vi "RP Test Scale.vi"() -> ()   [LabVIEW 2024]
uses:
  RP Calibration.ctl
  RP Calibration 4ch.ctl
  RP Channel Calibration.ctl
  RP Filter 4ch.ctl
  RP Channel Filter.ctl
  RP Calibration 2ch.ctl
panel:
  out "Scaled raw":dbl[][](graph)
  out "Unscaled":i16[][](graph)
  in  "ADC scale":dbl=8192.0
  out "Scaled":dbl[][](graph)
  in  "Channels":string[](array[string])=["V0", "V1"]
  in  "Unscaled data file":path=path "C:/Data/November_2024/111824/p004_111824.tdms"
  in  "RP Calibration":T1={"dataStructureId"=5, "wpCheck"=7, "fast_adc_count_1_1"=2, "padding"=0, "fast_adc_1_1"={"ch_0"={"baseScale"=1.0, "calibValue"=2837815, "offset"=-112, "padding 2"=0, "gainCalc"=1.0571686893755443}, "ch_1"={"baseScale"=1.0, "calibValue"=2835253, "offset"=-164, "padding 2"=0, "gainCalc"=1.056214269801971}, "ch_2"={"baseScale"=0.0, "calibValue"=0, "offset"=0, "padding 2"=0, "gainCalc"=0.0}, "ch_3"={"baseScale"=0.0, "calibValue"=0, "offset"=0, "padding 2"=0, "gainCalc"=0.0}}, "fast_adc_filter_1_1"={"ch_0"={"aa"=32147, "bb"=276423, "pp"=9830, "kk"=14260634}, "ch_1"={"aa"=32147, "bb"=276423, "pp"=9830, "kk"=14260634}, "ch_2"={"aa"=0, "bb"=0, "pp"=0, "kk"=0}, "ch_3"={"aa"=0, "bb"=0, "pp"=0, "kk"=0}}, "fast_adc_count_1_20"=2, "fast_adc_1_20"={"ch_0"={"baseScale"=1.0, "calibValue"=2666775, "offset"=-152, "padding 2"=0, "gainCalc"=0.9934513108181707}, "ch_1"={"baseScale"=1.0, "calibValue"=2664836, "offset"=-221, "padding 2"=0, "gainCalc"=0.9927289768786084}, "ch_2"={"baseScale"=0.0, "calibValue"=0, "offset"=0, "padding 2"=0, "gainCalc"=0.0}, "ch_3"={"baseScale"=0.0, "calibValue"=0, "offset"=0, "padding 2"=0, "gainCalc"=0.0}}, "fast_adc_filter_1_20"={"ch_0"={"aa"=16901, "bb"=193419, "pp"=9830, "kk"=14260634}, "ch_1"={"aa"=16901, "bb"=193419, "pp"=9830, "kk"=14260634}, "ch_2"={"aa"=0, "bb"=0, "pp"=0, "kk"=0}, "ch_3"={"aa"=0, "bb"=0, "pp"=0, "kk"=0}}, "fast_adc_count_1_1_ac"=0, "fast_adc_1_1_ac"={"ch_0"={"baseScale"=0.0, "calibValue"=0, "offset"=0, "padding 2"=0, "gainCalc"=0.0}, "ch_1"={"baseScale"=0.0, "calibValue"=0, "offset"=0, "padding 2"=0, "gainCalc"=0.0}, "ch_2"={"baseScale"=0.0, "calibValue"=0, "offset"=0, "padding 2"=0, "gainCalc"=0.0}, "ch_3"={"baseScale"=0.0, "calibValue"=0, "offset"=0, "padding 2"=0, "gainCalc"=0.0}}, "fast_adc_count_1_20_ac"=0, "fast_adc_1_20_ac"={"ch_0"={"baseScale"=0.0, "calibValue"=0, "offset"=0, "padding 2"=0, "gainCalc"=0.0}, "ch_1"={"baseScale"=0.0, "calibValue"=0, "offset"=0, "padding 2"=0, "gainCalc"=0.0}, "ch_2"={"baseScale"=0.0, "calibValue"=0, "offset"=0, "padding 2"=0, "gainCalc"=0.0}, "ch_3"={"baseScale"=0.0, "calibValue"=0, "offset"=0, "padding 2"=0, "gainCalc"=0.0}}, "fast_dac_count_x1"=2, "fast_dac_x1"={"ch_0"={"baseScale"=1.0, "calibValue"=2383506, "offset"=-287, "padding 2"=0, "gainCalc"=0.8879253630482418}, "ch_1"={"baseScale"=1.0, "calibValue"=2376551, "offset"=-279, "padding 2"=0, "gainCalc"=0.8853344231051493}}, "fast_dac_count_x5"=0, "fast_dac_x5"={"ch_0"={"baseScale"=0.0, "calibValue"=0, "offset"=0, "padding 2"=0, "gainCalc"=0.0}, "ch_1"={"baseScale"=0.0, "calibValue"=0, "offset"=0, "padding 2"=0, "gainCalc"=0.0}}}
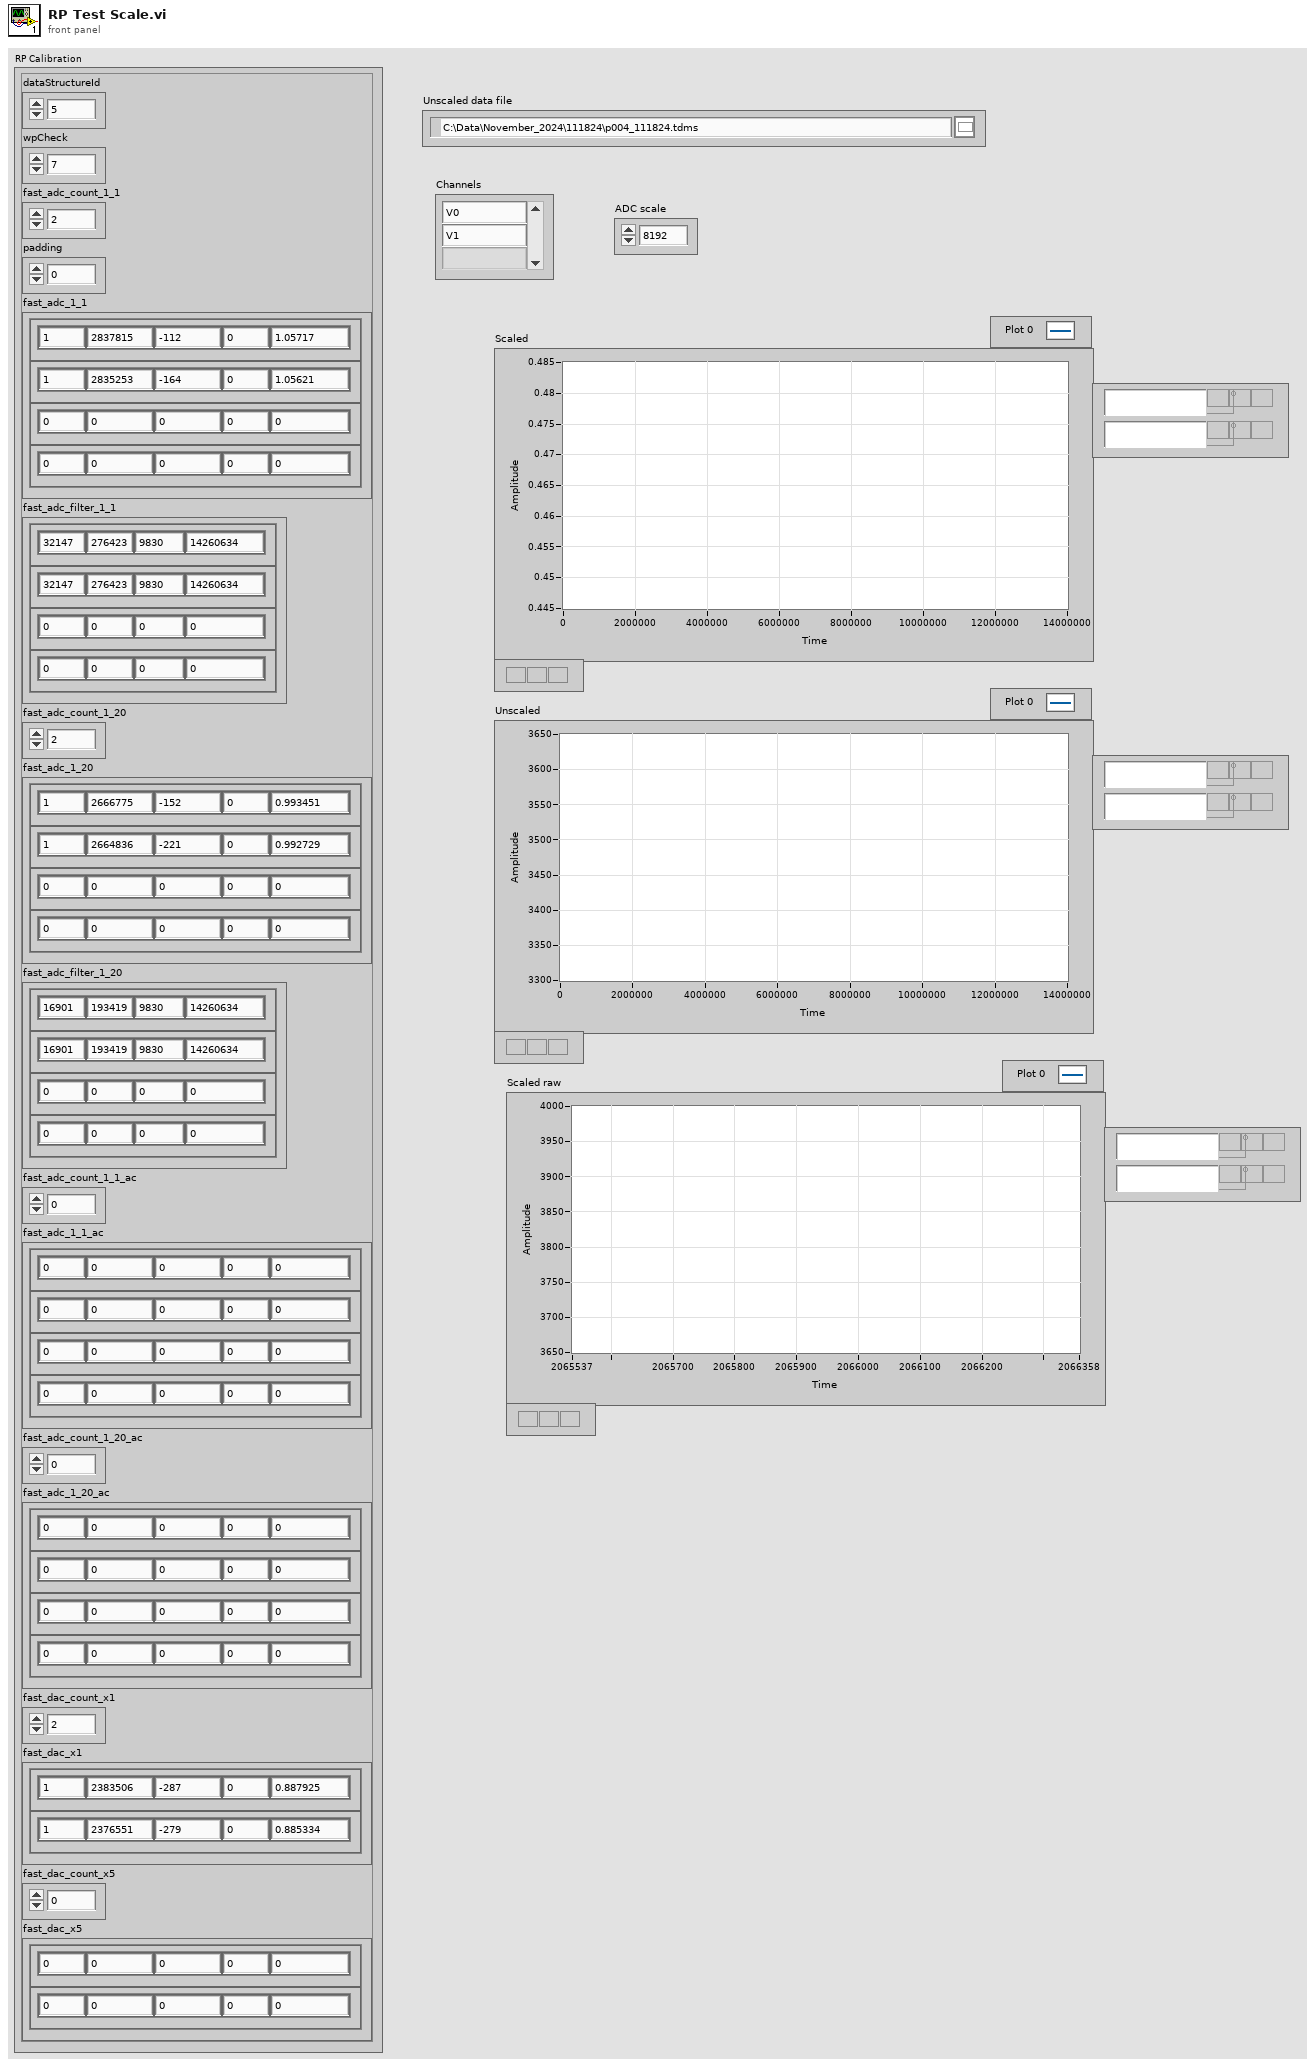
[diagram p1: front panel]
types:
  T1 = typedef "RP Calibration.ctl" = cluster{"dataStructureId":u8, "wpCheck":u8, "fast_adc_count_1_1":u16, "padding":u32, "fast_adc_1_1":T2, "fast_adc_filter_1_1":T4, "fast_adc_count_1_20":u64, "fast_adc_1_20":T2, "fast_adc_filter_1_20":T4, "fast_adc_count_1_1_ac":u64, "fast_adc_1_1_ac":T2, "fast_adc_count_1_20_ac":u64, "fast_adc_1_20_ac":T2, "fast_dac_count_x1":u64, "fast_dac_x1":T6, "fast_dac_count_x5":u64, "fast_dac_x5":T6}
  T2 = typedef "RP Calibration 4ch.ctl" = cluster{"ch_0":T3, "ch_1":T3, "ch_2":T3, "ch_3":T3}
  T3 = typedef "RP Channel Calibration.ctl" = cluster{"baseScale":sgl, "calibValue":u32, "offset":i32, "padding 2":i32, "gainCalc":dbl}
  T4 = typedef "RP Filter 4ch.ctl" = cluster{"ch_0":T5, "ch_1":T5, "ch_2":T5, "ch_3":T5}
  T5 = typedef "RP Channel Filter.ctl" = cluster{"aa":u32, "bb":u32, "pp":u32, "kk":u32}
  T6 = typedef "RP Calibration 2ch.ctl" = cluster{"ch_0":T3, "ch_1":T3}
  T7 = enum16{"open", "open or create", "create or replace", "create", "open (read-only)"}
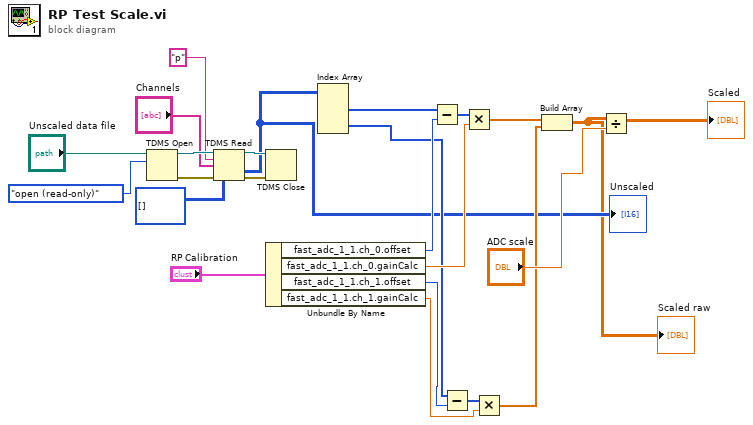
[diagram p0: block diagram]
diagram:
  n1 = TDMS Open(10:T7."open (read-only)" ("operation (0:open)"), 11:"Unscaled data file") -> (0:w21:errorcluster, 3:w22:refnum<k34>)  [unwired: 5 in]
  n2 = TDMS Read(0:w22, 5:"p" ("group name in"), 7:"Channels", 11:w21, 12:i16[][] []) -> (4:w17:refnum<k34>, 10:w2:i16[][], 15:w18:errorcluster)  [unwired: 3 in, 3 out]
  "Unscaled" <- w2
  n3 = TDMS Close(8:w18, 11:w17) -> ()  [unwired: 2 out]
  n4 = Unbundle By Name("RP Calibration") -> ("fast_adc_1_1.ch_0.offset"=w13:i32, "fast_adc_1_1.ch_0.gainCalc"=w11:dbl, "fast_adc_1_1.ch_1.offset"=w5:i32, "fast_adc_1_1.ch_1.gainCalc"=w4:dbl)
  n5 = Index Array(array=w2) -> (element #1=w14:i16[], element #2=w6:i16[])  [unwired: 4 in]
  n6 = Subtract(x=w14, y=w13) -> (x-y=w12:i32[])
  n7 = Subtract(x=w6, y=w5) -> (x-y=w7:i32[])
  n8 = Multiply(x=w12, y=w11) -> (x*y=w10:dbl[])
  n9 = Multiply(x=w7, y=w4) -> (x*y=w3:dbl[])
  n10 = Build Array(w10, w3) -> (w1:dbl[][])
  "Scaled raw" <- w1
  n11 = Divide(x=w1, y="ADC scale") -> (x/y=→"Scaled":dbl[][])
